vi "Main.vi"() -> ()   [LabVIEW 2015]
uses:
  controls/Names Selection.ctl
  controls/Status.ctl
  controls/Display.ctl
  controls/Names.ctl
  controls/Display Default.ctl
  <vilib>/Utility/miscctls.llb/LVRowAndColumnTypeDef.ctl
panel:
  in  "Write Note":bool
  in  "Reports":bool
  in  "Notes":string
  in  "Status":T1 items=["", "In", "Out", "Lunch", "Break"]
  in  "Name Selector":T2=20 caption="Name" items=["Adriana Chou", "Austin Scholp", "Boquan Liu", "Colin Schrof", "David Piotrowski", "Evan Polce", "Hayley Raj", "Hunter Bourne", "Hunter Huth", "Jack Ersbo", "Jack J", "Jacob Tangney", "Jake Reiss", "Jennifer German", "Jessica Wang", "JJ Lamb", "Lifan Yu", "Wyatt Barber", " "]
  in  "Admin Editing":bool
  in  "Update":bool
  in  "Exit":bool
  out "Display":string[][](table)
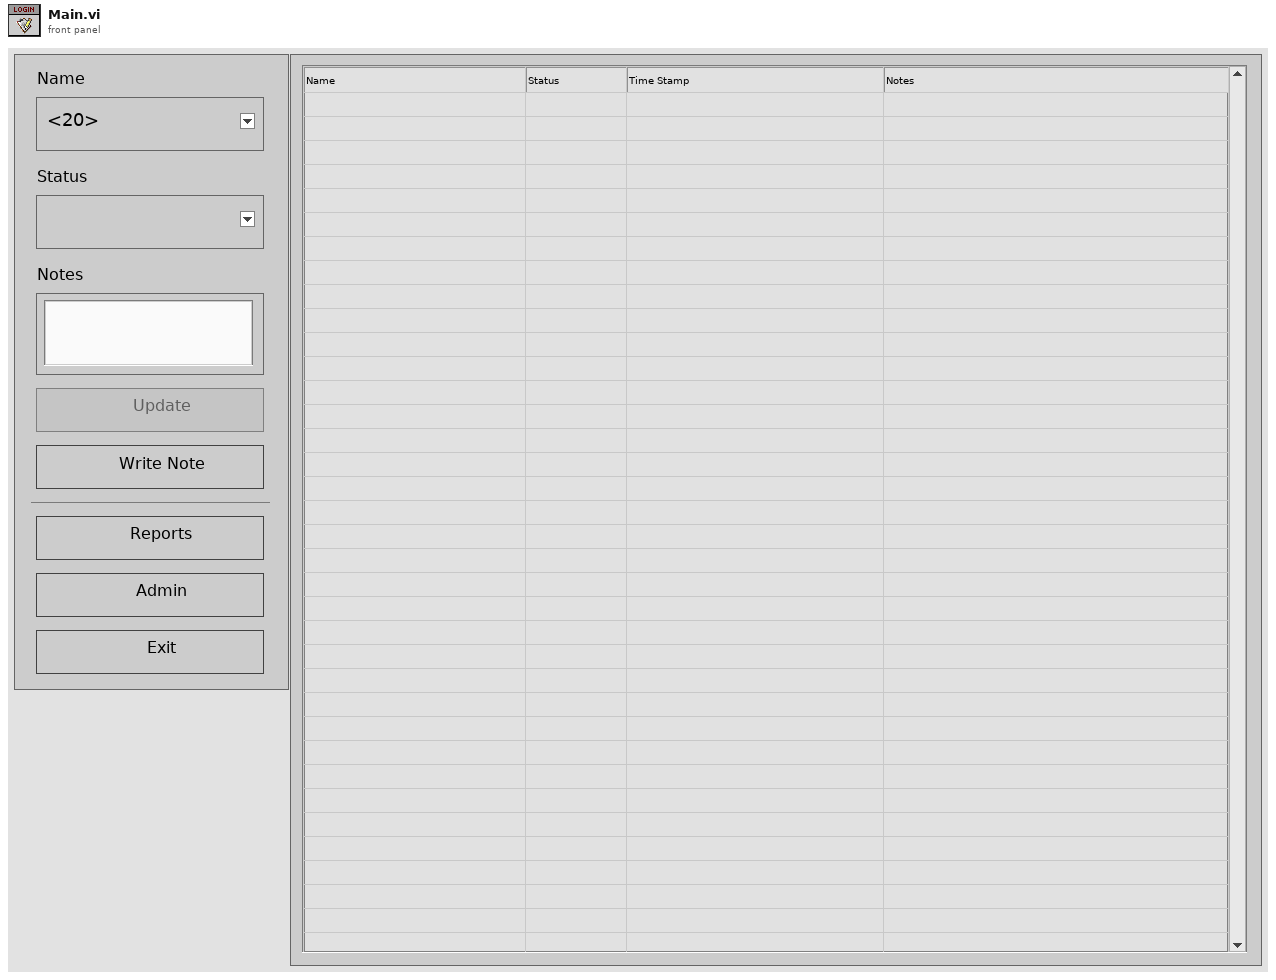
[diagram p1: front panel]
types:
  T1 = typedef "Status.ctl" = u16
  T2 = typedef "Names Selection.ctl" = u16
  T3 = typedef "Display.ctl" = cluster{"Name ":T4, "Status":T1, "Notes":string, "Display":T5}
  T4 = typedef "Names.ctl" = u16
  T5 = typedef "Display Default.ctl" = string[][]
  T6 = enum16{"open", "replace", "create", "open or create", "replace or create", "replace or create with confirmation"}
  T7 = enum8{"Enabled", "Disabled", "Disabled and Grayed Out"}
  T8 = typedef "LVRowAndColumnTypeDef.ctl" = cluster{"Row":i32, "Column":i32}
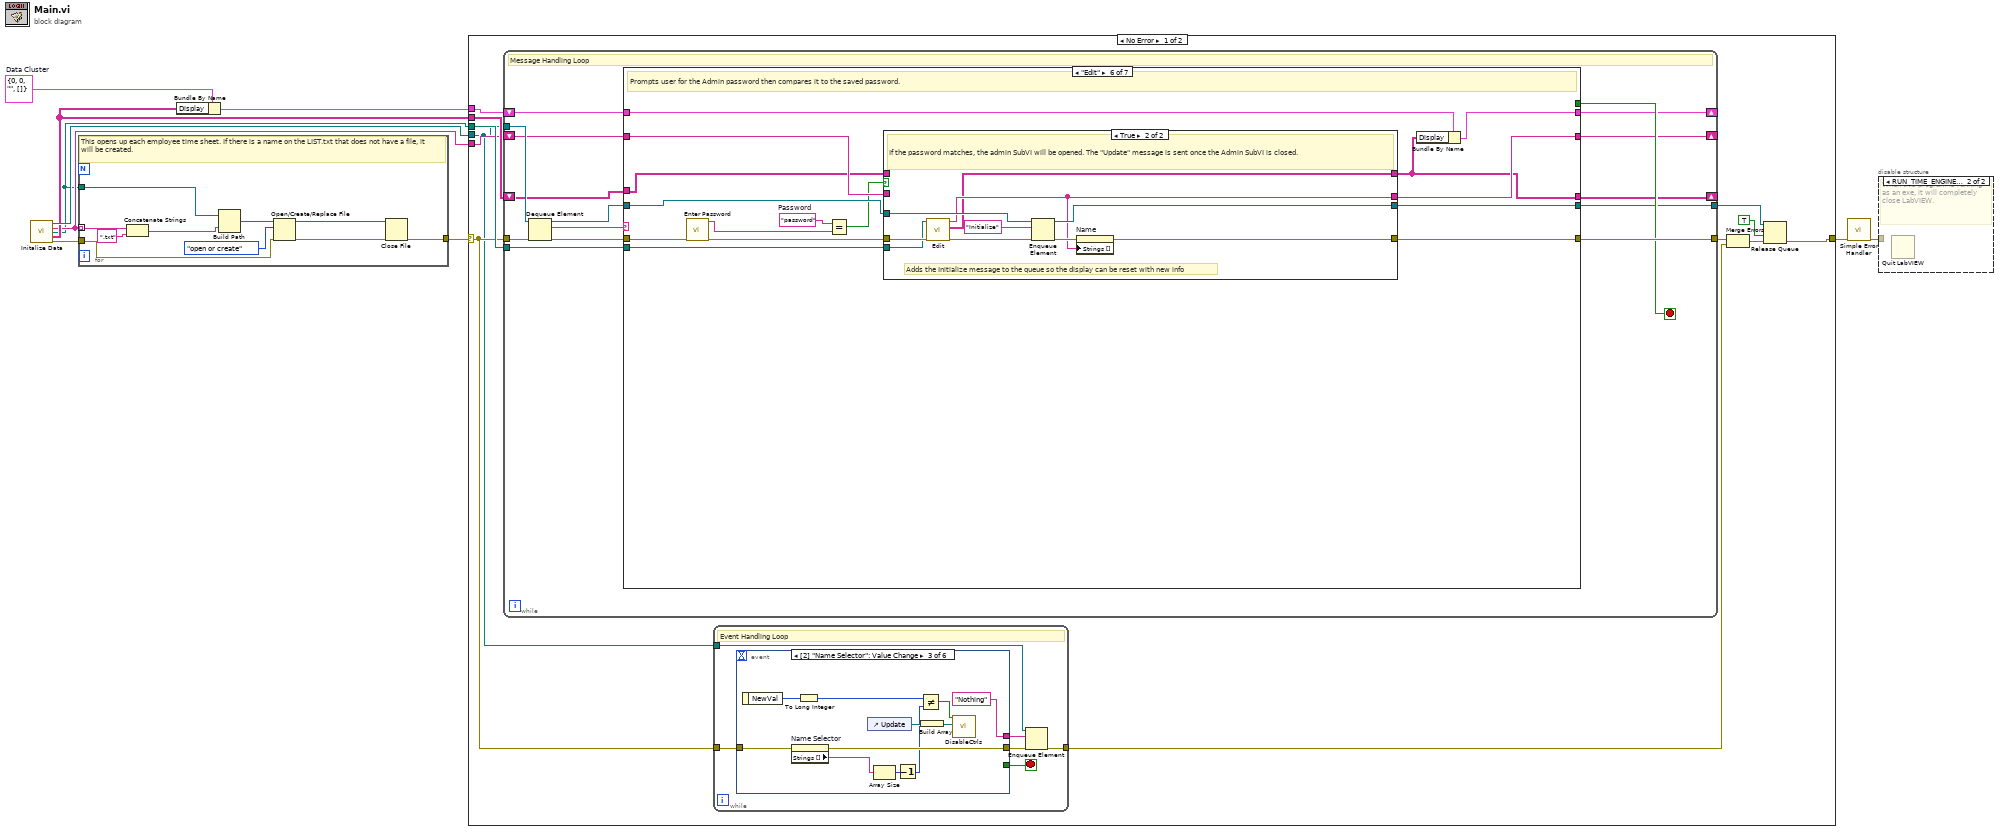
[diagram p0: block diagram]
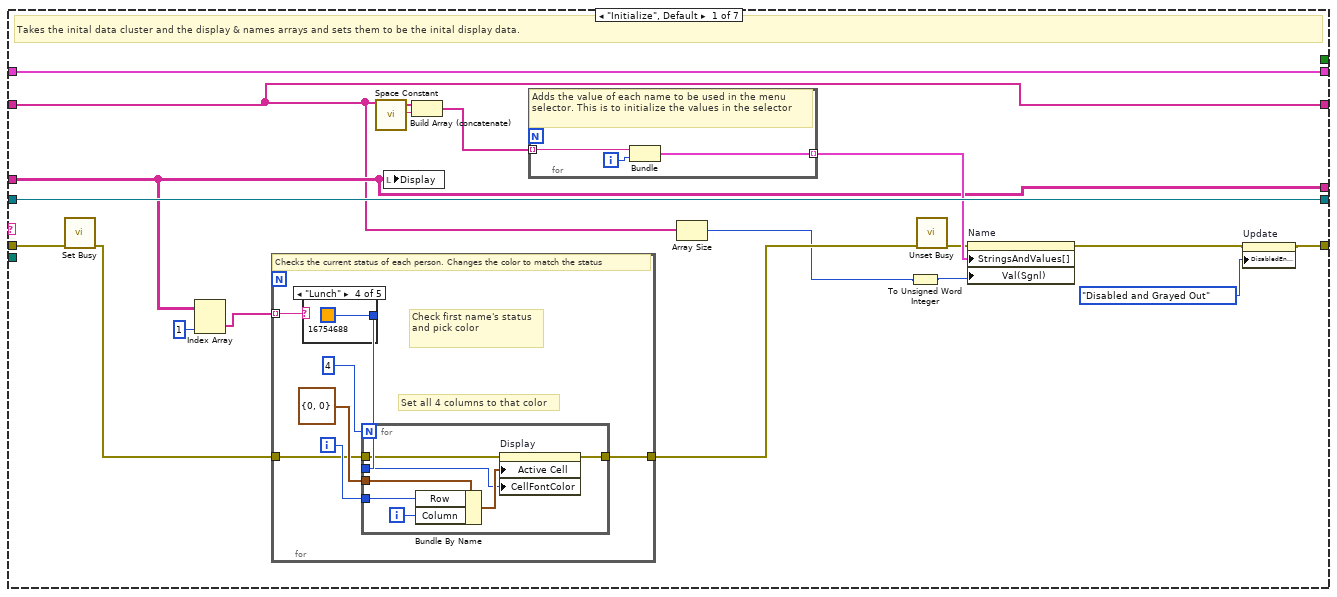
[diagram p2: hidden frame]
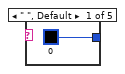
[diagram p3: hidden frame]
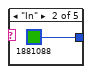
[diagram p4: hidden frame]
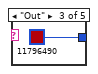
[diagram p5: hidden frame]
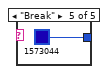
[diagram p6: hidden frame]
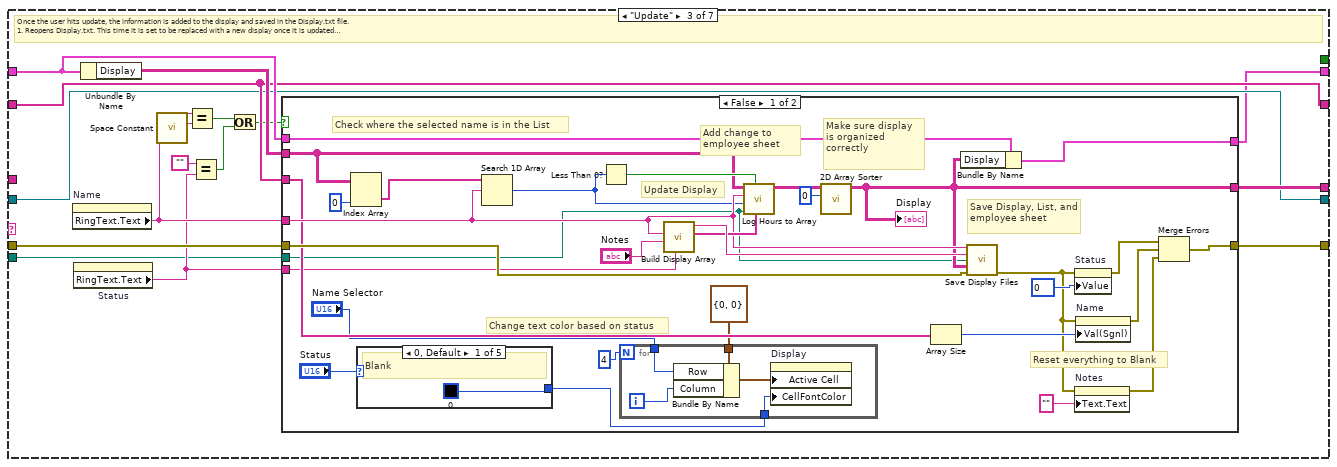
[diagram p8: hidden frame]
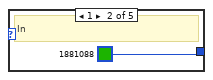
[diagram p9: hidden frame]
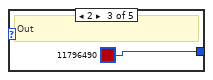
[diagram p10: hidden frame]
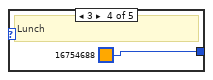
[diagram p11: hidden frame]
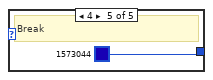
[diagram p12: hidden frame]
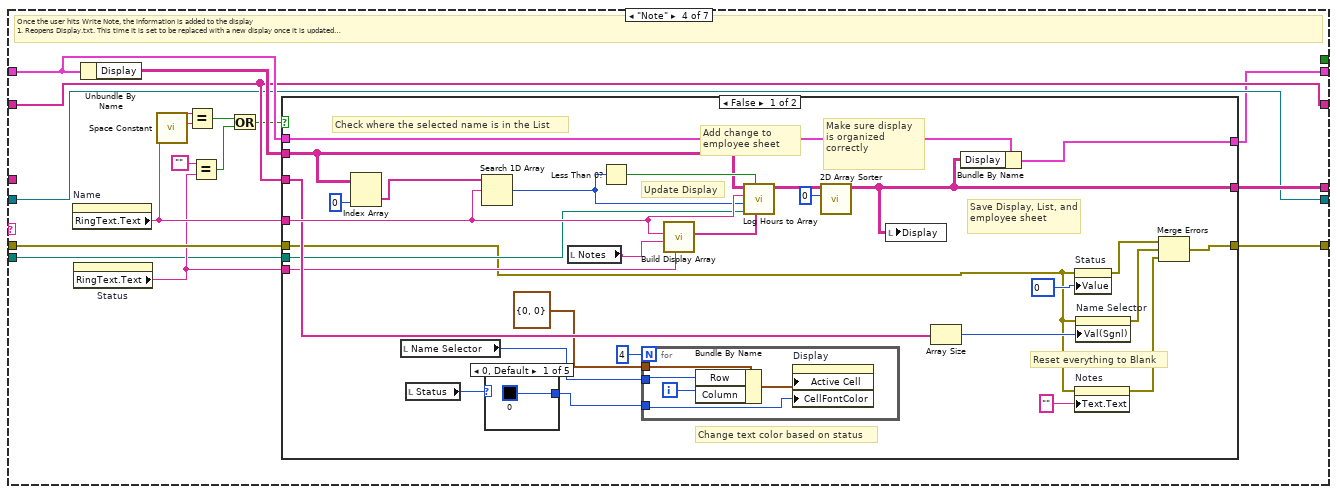
[diagram p14: hidden frame]
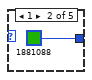
[diagram p15: hidden frame]
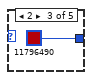
[diagram p16: hidden frame]
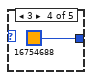
[diagram p17: hidden frame]
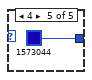
[diagram p18: hidden frame]
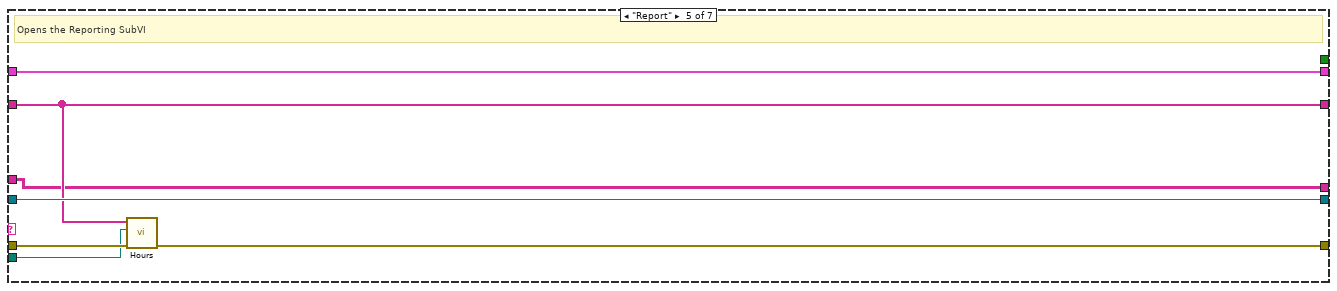
[diagram p20: hidden frame]
diagram:
  w9 = T3 {"Name "=0, "Status"=0, "Notes"="", "Display"=[]}  # Data Cluster
  n1 = call "Initalize Data.vi"() -> ("Queue out"=w10:refnum<queue>, "Names"=w3:string[], "VI or executable installation directory"=w1:path, "Display"=w4:string[][], "error out"=w5:errorcluster)  [unwired: 11 in]
  n2 = for {
    tunnel: w5 -> [w16]
    tunnel: [w12] -> w2
    tunnel: w3 -> [w15] mode=indexing
    tunnel: w1 -> [w11]
    # "This opens up each employee time sheet. If there is a name on the LIST.txt that does not have a file, it will be created."
    n3 = Concatenate Strings(w15, ".txt" ("string")) -> (w17:string)
    n4 = Build Path(base path=w11, name or relative path=w17) -> (appended path=w20:path)
    n5 = Open/Create/Replace File(file path (use dialog)=w20, error in=w16, operation (0:open)=T6."open or create") -> (refnum out=w13:refnum<file>, error out=w14:errorcluster)  [unwired: 3 in, 1 out]
    n6 = Close File(refnum=w13, error in=w14) -> (error out=w12:errorcluster)  [unwired: 1 out]
  }
  n7 = Bundle By Name(cluster=w9, "Display"=w4) -> (w8:T3)
  n8 = case shown="No Error" w2 {
    selector: w2 -> [w22 w283]
    tunnel: w10 -> [w21 _]
    tunnel: w8 -> [w28 _]
    tunnel: [w27 w283] -> w7
    tunnel: w4 -> [w26 _]
    tunnel: w3 -> [w23 _]
    tunnel: w1 -> [w24 _]
    frame No Error {
      n9 = while {
        tunnel: w21 -> [w47]
        tunnel: w22 -> [w46]
        tunnel: [w45] -> w32
        shift-right: [w41] -> _
        shift-left: w28 -> [w42]
        tunnel: [w39] -> w29
        shift-right: [w35] -> _
        shift-left: w23 -> [w36]
        shift-right: [w34] -> _
        shift-left: w26 -> [w37]
        tunnel: w24 -> [w33]
        stop <- w43 stop-if-true
        # "Message Handling Loop"
        n10 = Dequeue Element(queue=w47, error in (no error)=w46) -> (queue out=w40:refnum<queue>, element=w44:string, error out=w38:errorcluster)  [unwired: 1 in, 1 out]
        n11 = case shown="\"Edit\"" w44 {
          tunnel: [w52 w92 w106 w166 w215 w230 w250] -> w45
          tunnel: [_ _ _ _ _ _ TRUE] -> w43
          tunnel: w42 -> [w62 w88 w103 w163 w217 w224 w252]
          tunnel: [w62 w88 w100 w160 w217 w222 w252] -> w41
          tunnel: w40 -> [w65 w90 w101 w161 w216 w232 w251]
          tunnel: [w65 w90 w101 w161 w216 w231 w251] -> w39
          tunnel: w38 -> [w57 w92 w108 w168 w214 w219 w250]
          tunnel: w37 -> [w60 w91 _ _ w212 w225 w248]
          tunnel: w36 -> [w50 w89 w102 w162 w213 w227 w249]
          tunnel: [w50 w89 w102 w162 w213 w228 w249] -> w35
          tunnel: [w60 w91 w107 w167 w212 w223 w248] -> w34
          tunnel: w33 -> [_ _ w93 w153 w211 w221 _]
          frame "Initialize", Default {
            # "Takes the inital data cluster and the display & names arrays and sets them to be the inital display data."
            n12 = call <vilib>:"Set Busy.vi"("error in (no error)"=w57) -> ("error out"=w56:errorcluster)  [unwired: 9 in, 1 out]
            n13 = Index Array "Index Array"(array=w60, index (col)=1 ("disabled index (col)")) -> (element=w58:string[])  [unwired: 1 in]
            n14 = for {
              tunnel: [w70] -> w55
              tunnel: w58 -> [w69] mode=indexing
              tunnel: w56 -> [w66]
              i -> [w68]
              # "Set all 4 columns to that color"
              # "Check first name's status and pick color"
              # "Checks the current status of each person. Changes the color to match the status"
              n15 = case shown="\"Lunch\"" w69 {
                tunnel: [u32 0 ("Round Color Box") u32 1881088 ("Round Color Box") u32 11796490 ("Round Color Box") u32 16754688 ("Round Color Box") u32 1573044 ("Round Color Box")] -> w67
                frame " ", Default {
                  # "Blank"
                }
                frame "In" {
                  # "In"
                }
                frame "Out" {
                  # "Out"
                }
                frame "Lunch" {
                  # "Lunch"
                }
                frame "Break" {
                  # "Break"
                }
              }
              n16 = for {
                N: 4 -> [_]
                tunnel: T8 {"Row"=0, "Column"=0} ("Active Cell:Active Cell") -> [w79]
                tunnel: [w76] -> w70
                tunnel: w68 -> [w75]
                tunnel: w67 -> [w74]
                tunnel: w66 -> [w73]
                i -> [w78]
                n17 = Bundle By Name(cluster=w79, "Row"=w75, "Column"=w78) -> (w77:T8)
                n18 = property on="Display" class="Tbl (strict)"(error in=w73, "Active Cell"=w77, "CellFontColor"=w74) -> (error out=w76:errorcluster)  [unwired: 1 in, 1 out]
              }
            }
            n19 = call <vilib>:"Space Constant.vi"() -> ("String"=w64:string)
            n20 = local write "Display"(w60) -> ()
            n21 = Build Array (concatenate)(w50, w64) -> (w63:string[])
            n22 = for {
              tunnel: w63 -> [w87] mode=indexing
              tunnel: [w85] -> w61 mode=indexing
              i -> [w86]
              # "Adds the value of each name to be used in the menu selector. This is to initialize the values in the selector"
              n23 = Bundle("String"=w87, w86) -> (w85:cluster{"String":string, i32})  [unwired: 1 in]
            }
            n24 = Array Size(array=w50) -> (size(s)=w48:i32)
            n25 = To Unsigned Word Integer(number=w48) -> (unsigned 16bit integer=w49:u16)
            n26 = call <vilib>:"Unset Busy.vi"("error in (no error)"=w55) -> ("error out"=w54:errorcluster)  [unwired: 10 in]
            n27 = property on="Name" class="Ring (strict)"(error in=w54, "StringsAndValues[]"=w61, "Val(Sgnl)"=w49) -> (error out=w51:errorcluster)  [unwired: 1 in, 1 out]
            n28 = property on="Update" class="Bool"(error in=w51, "DisabledEnum"=T7."Disabled and Grayed Out" ("Disabled")) -> (error out=w52:errorcluster)  [unwired: 1 in, 1 out]
          }
          frame "Nothing" {
          }
          frame "Update" {
            # "Once the user hits update, the information is added to the display and saved in the Display.txt file.\n1. Reopens Display.txt. This time it is set to be replaced with a new display once it is updated\n2. Writes the new spreadsheet string data to the new Display.txt\n3. Closes Display.txt\n4. Finds the end of the employee data file\n5. Adds the new in/out data to the employee file"
            n29 = property on="Name" class="Ring (strict)"() -> ("RingText.Text"=w105:string)  [unwired: 2 in, 2 out]
            n30 = property on="Status" class="Ring (strict)"() -> ("RingText.Text"=w96:string)  [unwired: 2 in, 2 out]
            n31 = Unbundle By Name(w103) -> ("Display"=w104:T5)
            n32 = call <vilib>:"Space Constant.vi"() -> ("String"=w97:string)
            n33 = Equal?(x=w105, y=w97) -> (x = y?=w98:bool)
            n34 = Equal?(x="", y=w96) -> (x = y?=w95:bool)
            n35 = Or(x=w98, y=w95) -> (x .or. y?=w99:bool)
            n36 = case shown="False" w99 {
              tunnel: [w139 w151] -> w100
              tunnel: w103 -> [w131 w151]
              tunnel: w108 -> [w129 w152]
              tunnel: w102 -> [w124 _]
              tunnel: [w126 w150] -> w107
              tunnel: [w122 w152] -> w106
              tunnel: w105 -> [w130 _]
              tunnel: w104 -> [w128 w150]
              tunnel: w96 -> [w111 _]
              tunnel: w93 -> [w110 _]
              frame False {
                w132 = T1 0 items=["", "In", "Out", "Lunch", "Break"] ("Status")
                # "Save Display, List, and employee sheet"
                # "Reset everything to Blank"
                # "Update Display"
                # "Make sure display is organized correctly"
                # "Add change to employee sheet"
                # "Change text color based on status"
                # "Check where the selected name is in the List"
                n37 = Index Array "Index Array"(array=w128, index (col)=0 ("disabled index (col)")) -> (element=w125:string[])  [unwired: 1 in]
                n38 = case shown="0, Default" "Status" {
                  tunnel: [u32 0 ("Round Color Box") u32 1881088 ("Round Color Box") u32 11796490 ("Round Color Box") u32 16754688 ("Round Color Box") u32 1573044 ("Round Color Box")] -> w113
                  frame 0, Default {
                    # "Blank"
                  }
                  frame 1 {
                    # "In"
                  }
                  frame 2 {
                    # "Out"
                  }
                  frame 3 {
                    # "Lunch"
                  }
                  frame 4 {
                    # "Break"
                  }
                }
                n39 = Search 1D Array(1D array=w125, element=w130) -> (index of element=w114:i32)  [unwired: 1 in]
                n40 = Less Than 0?(x=w114) -> (x < 0?=w136:bool)
                n41 = for {
                  N: 4 -> [_]
                  tunnel: T8 {"Row"=0, "Column"=0} ("Active Cell:Active Cell") -> [w144]
                  tunnel: "Name Selector" -> [w142]
                  tunnel: w113 -> [w140]
                  i -> [w143]
                  n42 = Bundle By Name(cluster=w144, "Row"=w142, "Column"=w143) -> (w141:T8)
                  n43 = property on="Display" class="Tbl (strict)"("Active Cell"=w141, "CellFontColor"=w140) -> ()  [unwired: 2 in, 2 out]
                }
                n44 = call "Build Display Array.vi"("Status"=w111, "Notes"="Notes", "Name"=w130) -> ("Display Array"=w134:string[], "Spreadsheet String"=w137:string)  [unwired: 7 in]
                n45 = call "Log Hours to Array.vi"("Display Array"=w134, "Name doesn't exist?"=w136, "base path"=w110, "Name Index"=w114, "Name"=w130, "Display in"=w128) -> ("Display out"=w135:T5)  [unwired: 5 in]
                n46 = call "2D Array Sorter.vi"("Sorting Index"=0, "Array"=w135) -> ("sorted array"=w126:string[][])  [unwired: 8 in]
                "Display" <- w126
                n47 = Array Size(array=w124) -> (size(s)=w123:i32)
                n48 = Bundle By Name(cluster=w131, "Display"=w126) -> (w139:T3)
                n49 = call "Save Display Files.vi"("Name"=w130, "Spreadsheet String"=w137, "base path"=w110, "Display Array"=w126, "error in (no error)"=w129) -> ("error out"=w118:errorcluster)  [unwired: 10 in]
                n50 = property on="Status" class="Ring (strict)"(error in=w118, "Value"=w132) -> (error out=w119:errorcluster)  [unwired: 1 in, 1 out]
                n51 = property on="Notes" class="Str"(error in=w118, "Text.Text"="") -> (error out=w121:errorcluster)  [unwired: 1 in, 1 out]
                n52 = property on="Name" class="Ring (strict)"(error in=w118, "Val(Sgnl)"=w123) -> (error out=w120:errorcluster)  [unwired: 1 in, 1 out]
                n53 = Merge Errors(w119, w120, w121) -> (w122:errorcluster)
              }
              frame True {
              }
            }
          }
          frame "Note" {
            # "Once the user hits Write Note, the information is added to the display \n1. Reopens Display.txt. This time it is set to be replaced with a new display once it is updated\n2. Writes the new spreadsheet string data to the new Display.txt\n3. Closes Display.txt\n4. Finds the end of the employee data file\n5. Adds the new in/out data to the employee file"
            n54 = property on="Name" class="Ring (strict)"() -> ("RingText.Text"=w165:string)  [unwired: 2 in, 2 out]
            n55 = property on="Status" class="Ring (strict)"() -> ("RingText.Text"=w156:string)  [unwired: 2 in, 2 out]
            n56 = Unbundle By Name(w163) -> ("Display"=w164:T5)
            n57 = call <vilib>:"Space Constant.vi"() -> ("String"=w157:string)
            n58 = Equal?(x=w165, y=w157) -> (x = y?=w158:bool)
            n59 = Equal?(x="", y=w156) -> (x = y?=w155:bool)
            n60 = Or(x=w158, y=w155) -> (x .or. y?=w159:bool)
            n61 = case shown="False" w159 {
              tunnel: [w197 w209] -> w160
              tunnel: w163 -> [w191 w209]
              tunnel: w168 -> [w175 w210]
              tunnel: w162 -> [w186 _]
              tunnel: [w174 w208] -> w167
              tunnel: [w184 w210] -> w166
              tunnel: w165 -> [w190 _]
              tunnel: w164 -> [w189 w208]
              tunnel: w156 -> [w179 _]
              tunnel: w153 -> [w178 _]
              frame False {
                w192 = T1 0 items=["", "In", "Out", "Lunch", "Break"] ("Status")
                # "Change text color based on status"
                # "Save Display, List, and employee sheet"
                # "Reset everything to Blank"
                # "Update Display"
                # "Make sure display is organized correctly"
                # "Add change to employee sheet"
                # "Check where the selected name is in the List"
                n62 = Index Array "Index Array"(array=w189, index (col)=0 ("disabled index (col)")) -> (element=w187:string[])  [unwired: 1 in]
                n63 = local read "Name Selector"() -> (w170:T2)
                n64 = local read "Status"() -> (w171:T1)
                n65 = Search 1D Array(1D array=w187, element=w190) -> (index of element=w180:i32)  [unwired: 1 in]
                n66 = case shown="0, Default" w171 {
                  tunnel: [u32 0 ("Round Color Box") u32 1881088 ("Round Color Box") u32 11796490 ("Round Color Box") u32 16754688 ("Round Color Box") u32 1573044 ("Round Color Box")] -> w169
                  frame 0, Default {
                    # "Blank"
                  }
                  frame 1 {
                    # "In"
                  }
                  frame 2 {
                    # "Out"
                  }
                  frame 3 {
                    # "Lunch"
                  }
                  frame 4 {
                    # "Break"
                  }
                }
                n67 = local read "Notes"() -> (w176:string)
                n68 = Less Than 0?(x=w180) -> (x < 0?=w196:bool)
                n69 = for {
                  N: 4 -> [_]
                  tunnel: T8 {"Row"=0, "Column"=0} ("Active Cell:Active Cell") -> [w207]
                  tunnel: w170 -> [w205]
                  tunnel: w169 -> [w203]
                  i -> [w206]
                  n70 = Bundle By Name(cluster=w207, "Row"=w205, "Column"=w206) -> (w204:T8)
                  n71 = property on="Display" class="Tbl (strict)"("Active Cell"=w204, "CellFontColor"=w203) -> ()  [unwired: 2 in, 2 out]
                }
                n72 = call "Build Display Array.vi"("Status"=w179, "Notes"=w176, "Name"=w190) -> ("Display Array"=w194:string[])  [unwired: 7 in, 1 out]
                n73 = call "Log Hours to Array.vi"("Display Array"=w194, "Name doesn't exist?"=w196, "base path"=w178, "Name Index"=w180, "Name"=w190, "Display in"=w189) -> ("Display out"=w195:T5)  [unwired: 5 in]
                n74 = call "2D Array Sorter.vi"("Sorting Index"=0, "Array"=w195) -> ("sorted array"=w174:string[][])  [unwired: 8 in]
                n75 = local write "Display"(w174) -> ()
                n76 = Array Size(array=w186) -> (size(s)=w185:i32)
                n77 = Bundle By Name(cluster=w191, "Display"=w174) -> (w197:T3)
                n78 = property on="Status" class="Ring (strict)"(error in=w175, "Value"=w192) -> (error out=w181:errorcluster)  [unwired: 1 in, 1 out]
                n79 = property on="Notes" class="Str"(error in=w175, "Text.Text"="") -> (error out=w183:errorcluster)  [unwired: 1 in, 1 out]
                n80 = property on="Name Selector" class="Ring (strict)"(error in=w175, "Val(Sgnl)"=w185) -> (error out=w182:errorcluster)  [unwired: 1 in, 1 out]
                n81 = Merge Errors(w181, w182, w183) -> (w184:errorcluster)
              }
              frame True {
              }
            }
          }
          frame "Report" {
            # "Opens the Reporting SubVI"
            n82 = call "Hours.vi"("error in (no error)"=w214, "base path"=w211, "Names"=w213) -> ("error out"=w215:errorcluster)  [unwired: 8 in]
          }
          frame "Edit" {
            w229 = "password"  # Password
            # "Prompts user for the Admin password then compares it to the saved password."
            n83 = call "Enter Password.vi"("Error In"=w219) -> ("Error Out"=w220:errorcluster, "Password Out"=w218:string)  [unwired: 9 in]
            n84 = Equal?(x=w229, y=w218) -> (x = y?=w226:bool)
            n85 = case shown="True" w226 {
              tunnel: w232 -> [w237 w247]
              tunnel: [w237 w245] -> w231
              tunnel: [w235 w241] -> w230
              tunnel: w220 -> [w236 w243]
              tunnel: [w234 w240] -> w228
              tunnel: w227 -> [w234 _]
              tunnel: [w233 w239] -> w223
              tunnel: w225 -> [w233 _]
              tunnel: w221 -> [_ w238]
              frame False {
                # "If the password does not match, a message will be displayed"
                n86 = call "Display Message to User"("error in (no error)"=w236) -> ("error out"=w235:errorcluster)  [unwired: 9 in, 1 out]
              }
              frame True {
                # "Adds the Initialize message to the queue so the display can be reset with new info"
                # "If the password matches, the admin SubVI will be opened. The \"Update\" message is sent once the Admin SubVI is closed."
                n87 = call "Edit.vi"("error In"=w243, "base path"=w238) -> ("error out"=w246:errorcluster, "New Display"=w239:string[][], "Names List"=w240:string[])  [unwired: 7 in]
                n88 = Enqueue Element(queue=w247, element="Initialize", error in (no error)=w246) -> (queue out=w245:refnum<queue>, error out=w242:errorcluster)  [unwired: 1 in, 1 out]
                n89 = property on="Name" class="Ring (strict)"(error in=w242, "Strings []"=w240) -> (error out=w241:errorcluster)  [unwired: 1 in, 1 out]
              }
            }
            n90 = Bundle By Name(cluster=w224, "Display"=w223) -> (w222:T3)
          }
          frame "Exit" {
            # "Once the \"exit\" message is received, this loop will be stopped."
          }
        }
      }
      n91 = while {
        tunnel: w21 -> [w258]
        tunnel: w22 -> [w255]
        tunnel: [w254] -> w31
        stop <- w259 stop-if-true
        # "Event Handling Loop"
        n92 = event shown="[2] \"Name Selector\": Value Change" {
          selector: _ -> [_ _ _ _ _ _]
          dyn-events: _ -> [_ _ _ _ _ _]
          timeout: _ -> [_ _ _ _ _ _]
          tunnel: [_ FALSE _ _ _ TRUE] -> w259
          tunnel: ["Update" "Note" "Nothing" "Report" "Edit" "Exit"] -> w257
          tunnel: [w260 w263 w267 w276 w278 w280] -> w256
          tunnel: w255 -> [w260 w263 w268 w276 w278 w280]
          event "Update": Value Change {
            # "Sends the \"Update\" message when the update button is pressed"
            n93 = event-data() -> ()  [unwired: 1 in, 1 out]
          }
          event "Write Note": Value Change {
            n94 = event-data() -> ()  [unwired: 1 in, 1 out]
          }
          event Value Change {
            n95 = event-data() -> ("NewVal"=w271:T2)  [unwired: 1 in]
            n96 = property on="Name Selector" class="Ring (strict)"(error in=w268) -> (error out=w267:errorcluster, "Strings []"=w269:string[])  [unwired: 1 in, 1 out]
            n97 = To Long Integer(number=w271) -> (32bit integer=w270:i32)
            n98 = control-ref of="Update"() -> (w275:refnum<vi>)
            n99 = Array Size(array=w269) -> (size(s)=w266:i32)
            n100 = Decrement(x=w266) -> (x-1=w265:i32)
            n101 = Not Equal?(x=w270, y=w265) -> (x != y?=w272:bool)
            n102 = Build Array(w275) -> (w274:refnum<vi>[])
            n103 = call "DisableCtrls.vi"("Array"=w274, "Enabled?"=w272) -> ()  [unwired: 10 in]
          }
          event "Reports": Value Change {
            # "Sends the \"Report\" message when the reports button is pressed"
            n104 = event-data() -> ()  [unwired: 1 in, 1 out]
          }
          event "Admin Editing": Value Change {
            # "Sends the \"Edit\" meesage when the Admin button is pressed"
            n105 = event-data() -> ()  [unwired: 1 in, 1 out]
          }
          event "Exit": Value Change {
            # "Sends the \"Exit\" message when the Exit button is pressed. It also stops the event handling loop"
            n106 = event-data() -> ()  [unwired: 1 in, 1 out]
          }
        }
        n107 = Enqueue Element(queue=w258, element=w257, error in (no error)=w256) -> (error out=w254:errorcluster)  [unwired: 1 in, 2 out]
      }
      n108 = Merge Errors(w32, w31) -> (w25:errorcluster)
      n109 = Release Queue(queue=w29, force destroy? (F)=TRUE, error in (no error)=w25) -> (error out=w27:errorcluster)  [unwired: 2 out]
    }
    frame Error {
    }
  }
  n110 = call <vilib>:"Simple Error Handler.vi"("error in (no error)"=w7) -> ("error out"=w6:errorcluster)  [unwired: 4 in, 4 out]
  n111 = disable-structure shown="RUN_TIME_ENGINE==True" {
    disable-tunnel: w6 -> [_ _]
    frame condition #0 (active) {
    }
    frame condition #1 {
      # "When this program is running as an exe, it will completely close LabVIEW."
      n112 = Quit LabVIEW() -> ()  [unwired: 1 in]
    }
  }
